vi "getSlitWidth.vi"(8 "error in (no error)":errorcluster, 9 "Monochromator in":refnum<class "Monochromator.lvclass">, 10 "SlitType in":T2, 11 "MonoState in":refnum<class "MonoState.lvclass">) -> (0 "error out":errorcluster, 1 "Monochromator out":refnum<class "Monochromator.lvclass">, 2 "position":T1, 3 "MonoState out":refnum<class "MonoState.lvclass">)   [LabVIEW 2016, in "MonoState.lvclass"]
uses:
  MonoState.lvclass
  Typedefs/SlitType.ctl
  Typedefs/slit.ctl
  Typedefs/slitWidth.ctl
  Monochromator/Monochromator.lvclass
  Monochromator/Monochromator.lvclass/Monochromator.ctl
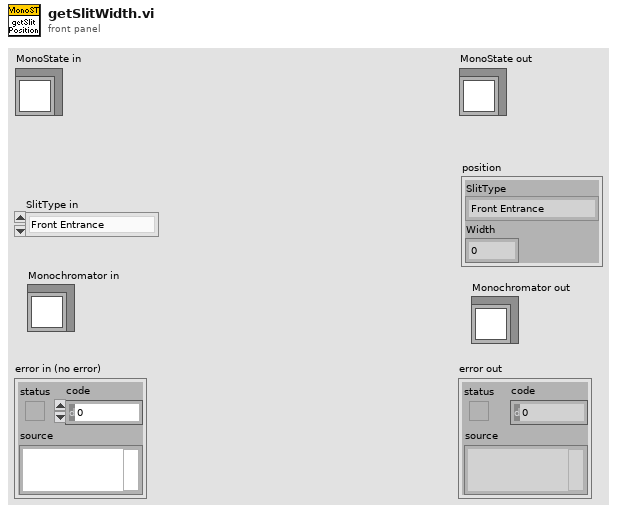
[diagram p1: front panel]
types:
  T1 = typedef "slit.ctl" = cluster{"SlitType":T2, "Width":T3}
  T2 = typedef "SlitType.ctl" = enum16{"Front Entrance", "Side Entrance", "Front Exit", "Side Exit", "First Intermediate", "Second Intermediate"}
  T3 = typedef "slitWidth.ctl" = dbl
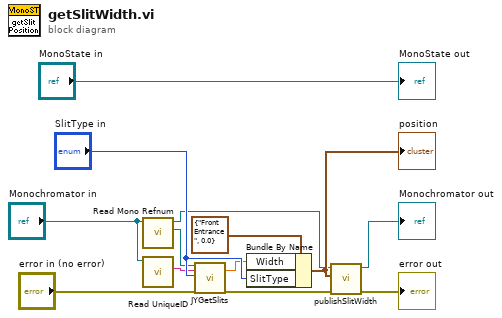
[diagram p0: block diagram]
diagram:
  n1 = call "Read Mono Refnum.vi"("Monochromator in"="Monochromator in") -> ("Mono Refnum"=w3:refnum<k7>, "Monochromator out"=w2:refnum<class "Monochromator.lvclass">)  [unwired: 8 in, 1 out]
  n2 = call "Read UniqueID.vi"("Monochromator in"="Monochromator in") -> ("UniqueID"=w1:string)  [unwired: 8 in, 2 out]
  n3 = call "JYGetSlits.vi"("MonoRefNum IN"=w3, "UniqueID"=w1, "Slit"="SlitType in", "error in (no error)"="error in (no error)") -> ("Slit Width"=w5:dbl, "error out"=w6:errorcluster)  [unwired: 12 in, 2 out]
  n4 = Bundle By Name(cluster=T1 {"SlitType"=enum."Front Entrance", "Width"=0.0} ("position 2"), "Width"=w5, "SlitType"="SlitType in") -> (w8:T1)
  "position" <- w8
  n5 = call "publishSlitWidth.vi"("error in (no error)"=w6, "slitPosition"=w8, "Monochromator in"=w2) -> ("error out"=→"error out":errorcluster, "Monochromator out"=→"Monochromator out":refnum<class "Monochromator.lvclass">)  [unwired: 7 in]
  "MonoState out" <- "MonoState in"
